vi "analyse.vi"(8 "error in (no error)":errorcluster, 11 "TrajectoryDL091126GenericVoxel in":refnum<class "TrajectoryDL091126GenericVoxel.lvclass">) -> (0 "error out":errorcluster, 3 "TrajectoryDL091126GenericVoxel out":refnum<class "TrajectoryDL091126GenericVoxel.lvclass">)   [LabVIEW 2010, in "TrajectoryDL091126GenericVoxel.lvclass"]
uses:
  TrajectoryDL091126GenericVoxel.lvclass
  common/classes/ImageCollection/ImageCollection/ImageCollection.lvclass
  common/enumerations/x_y_z_enumeration.ctl
  common/enumerations/functional_global_action_enum.ctl
  common/classes/ImageCollection/ImageCollection/add_mode_enum.ctl
  common/classes/Image/Image/Image.lvclass
  common/classes/ErrorController/ErrorController/class_data.vi
  <vilib>/vision/NI_Vision_Development_Module.lvlib
  common/classes/ErrorController/ErrorController/ErrorController.lvclass
panel:
  in  "loadZPositionDataButton":bool
  in  "loadYPositionDataButton":bool
  out "y signals 2":dbl[][](graph)
  in  "position scale z":dbl(slide) scale=0.0..20000.0
  in  "position scale y":dbl(slide) scale=0.0..20000.0
  out "y signals":dbl[][](graph)
  in  "position scale x":dbl(slide) scale=0.0..20000.0
  in  "defineTrajectoryButton":bool
  in  "line":i32(slide) scale=0.0..10.0
  out "x signals":dbl[][](graph)
  in  "doneButton":bool
  in  "loadXPositionDataButton":bool
  # "Analyse position feedback"
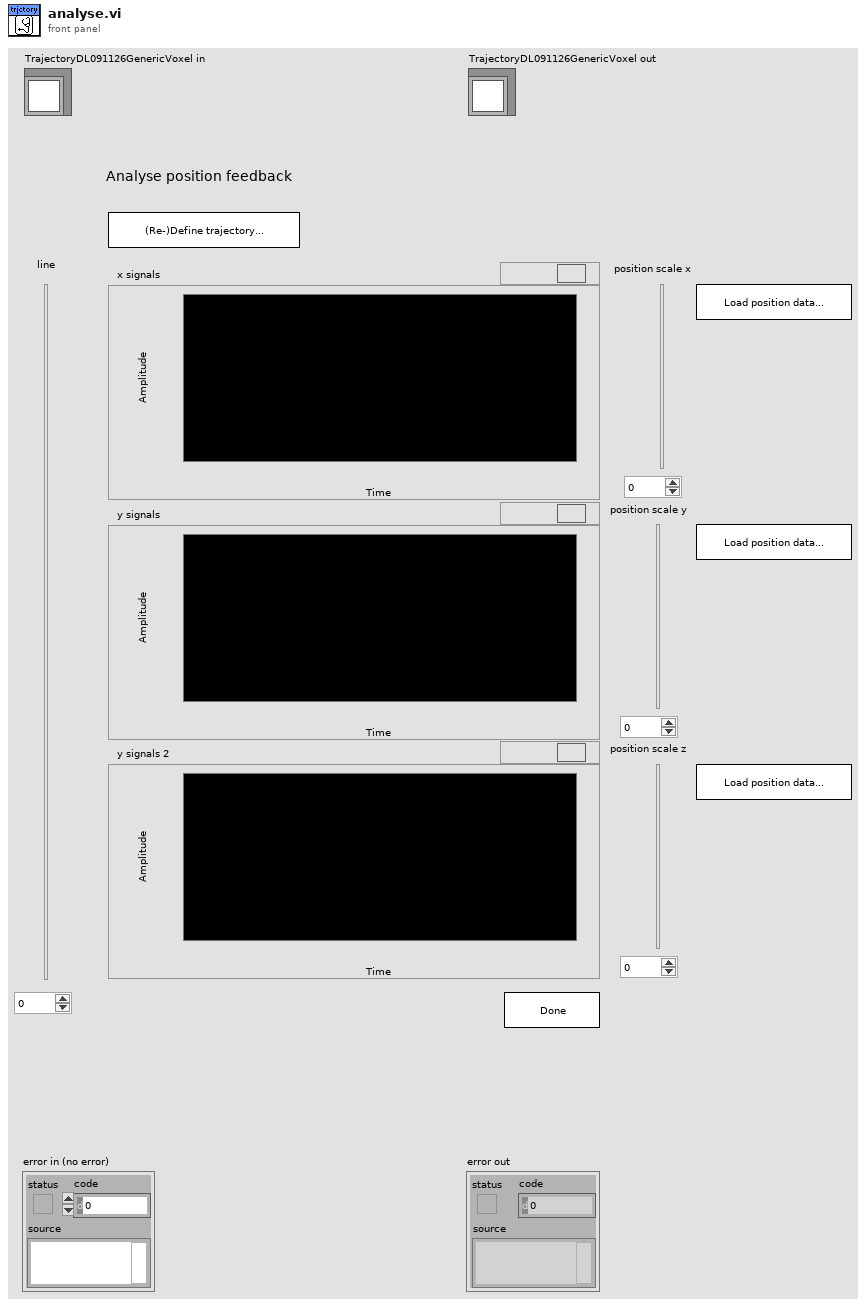
[diagram p1: front panel]
types:
  T1 = typedef "x_y_z_enumeration.ctl" = enum16{"x", "y", "z"}
  T2 = typedef "Image Type" = u32
  T3 = typedef "functional_global_action_enum.ctl" = enum16{"get", "set", "reset"}
  T4 = typedef "ImageCollection.lvclass/add_mode_enum.ctl" = enum16{"instance", "copy"}
  T5 = typedef "IMAQ Image.ctl" = refnum<image>
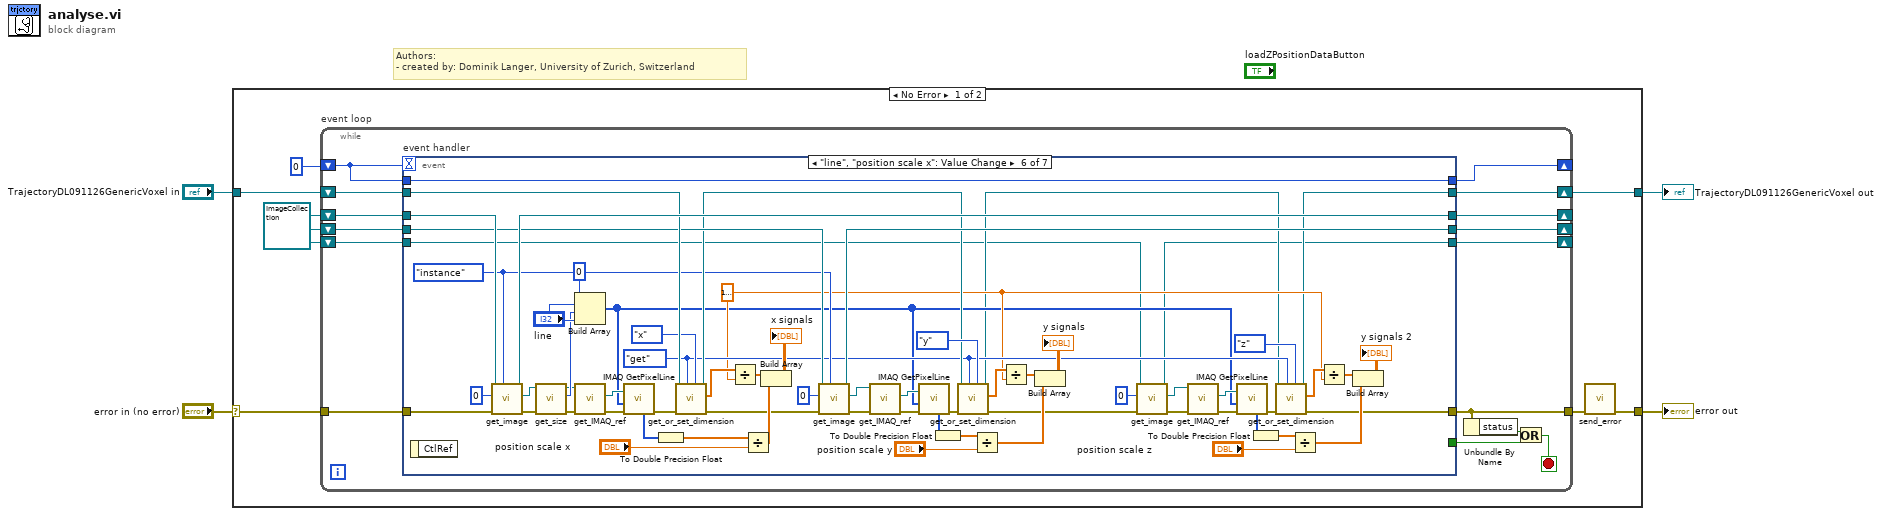
[diagram p0: block diagram]
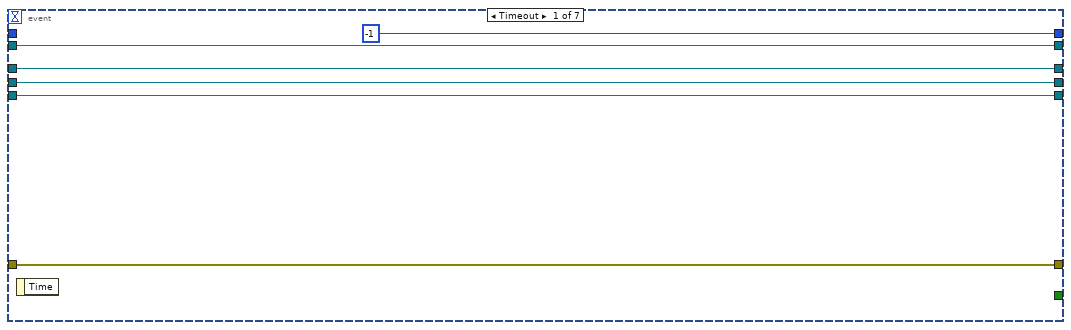
[diagram p2: hidden frame]
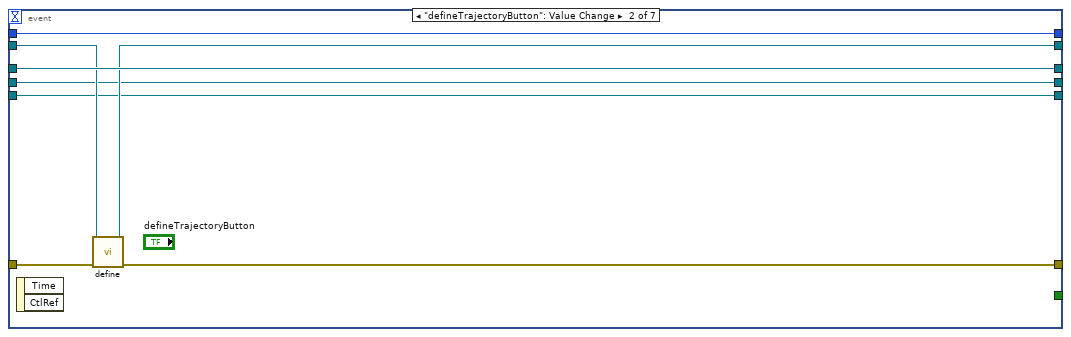
[diagram p3: hidden frame]
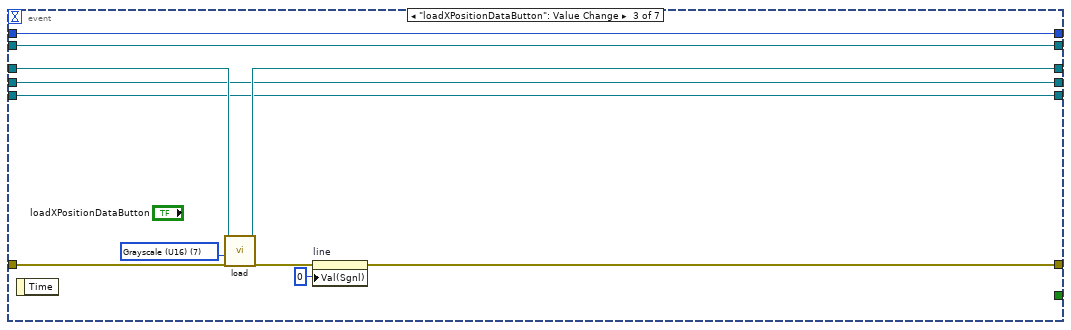
[diagram p4: hidden frame]
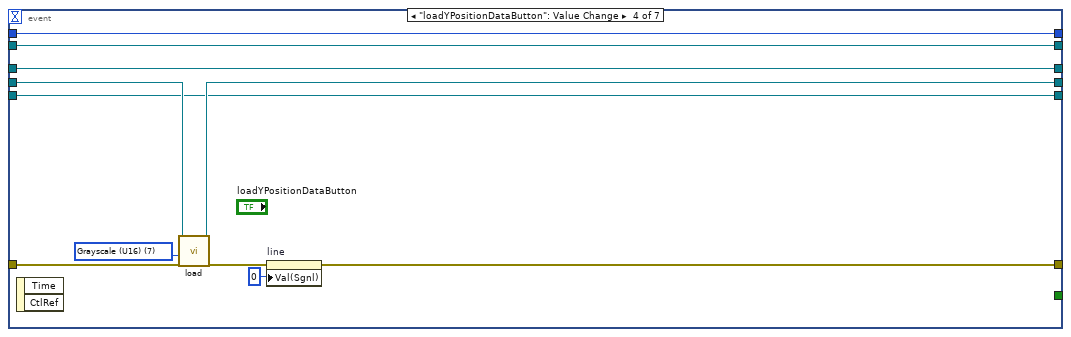
[diagram p5: hidden frame]
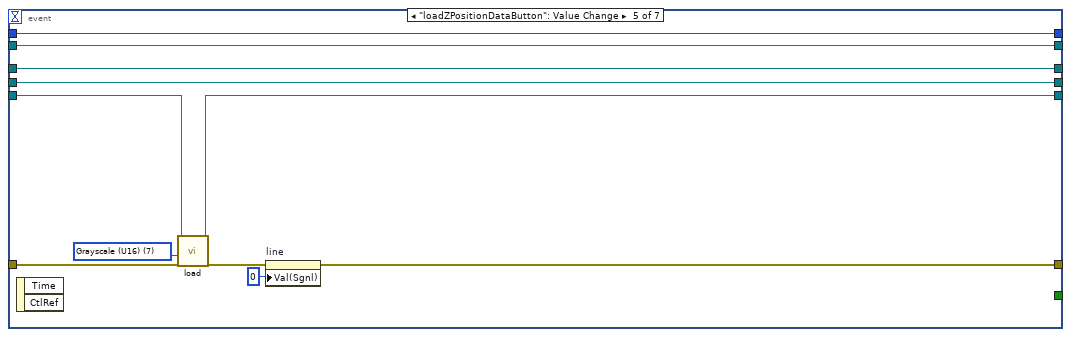
[diagram p6: hidden frame]
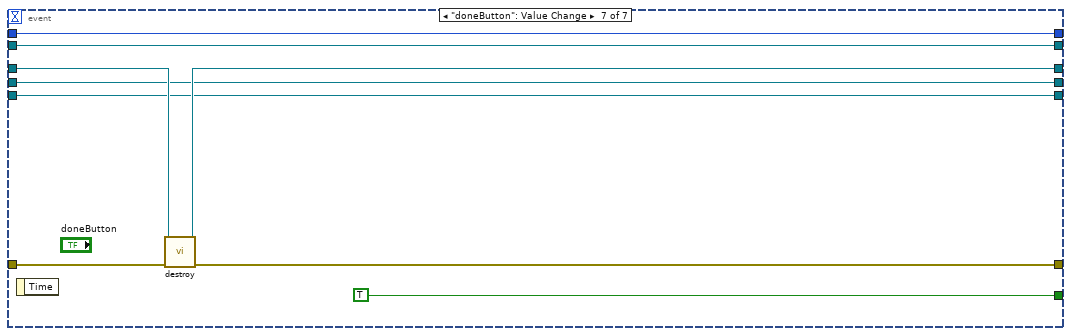
[diagram p7: hidden frame]
diagram:
  # "Authors: \n- created by: Dominik Langer, University of Zurich, Switzerland"
  n1 = case shown="No Error" "error in (no error)" {
    selector: "error in (no error)" -> [w11 w150]
    tunnel: [w5 w150] -> w3
    tunnel: [w9 w149] -> w1
    tunnel: "TrajectoryDL091126GenericVoxel in" -> [w10 w149]
    frame No Error {
      w7 = refnum<class "ImageCollection.lvclass"> refnum ("ImageCollection.lvclass")
      n2 = while "event loop" {
        shift-right: [w25] -> w9
        shift-left: w10 -> [w26]
        shift-right: [w18] -> _
        shift-left: w7 -> [w19]
        shift-right: [w16] -> _
        shift-left: 0 -> [w17]
        shift-right: [w13] -> _
        shift-left: w7 -> [w15]
        shift-right: [w12] -> _
        shift-left: w7 -> [w14]
        tunnel: w11 -> [w24]
        tunnel: [w23] -> w6
        stop <- w22 stop-if-true
        n3 = event "event handler" shown="[5] \"line\", \"position scale x \": Value Change" {
          selector: _ -> [_ _ _ _ _ _ _]
          dyn-events: _ -> [_ _ _ _ _ _ _]
          timeout: w17 -> [_ _ _ _ _ _ _]
          tunnel: w26 -> [w32 w36 w51 w62 w73 w124 w148]
          tunnel: [w32 w35 w51 w62 w73 w76 w148] -> w25
          tunnel: w24 -> [w29 w39 w50 w55 w64 w139 w144]
          tunnel: [w29 w38 w45 w54 w63 w82 w143] -> w23
          tunnel: [_ _ _ _ _ _ TRUE] -> w21
          tunnel: [w30 w37 w48 w61 w72 w136 w145] -> w18
          tunnel: w19 -> [w30 w37 w49 w61 w72 w137 w146]
          tunnel: [-1 w40 w43 w60 w71 w126 w142] -> w16
          tunnel: w17 -> [_ w40 w43 w60 w71 w126 w142]
          tunnel: w15 -> [w28 w34 w42 w56 w70 w108 w141]
          tunnel: w14 -> [w27 w33 w41 w52 w66 w75 w140]
          tunnel: [w28 w34 w42 w53 w70 w107 w141] -> w13
          tunnel: [w27 w33 w41 w52 w65 w74 w140] -> w12
          event Timeout {
            n4 = event-data() -> ()  [unwired: 1 in, 1 out]
          }
          event "defineTrajectoryButton": Value Change {
            n5 = event-data() -> ()  [unwired: 1 in, 2 out]
            n6 = call-dynamic "define.vi"("error in (no error)"=w39, "GenericTrajectory in"=w36) -> ("error out"=w38:errorcluster, "GenericTrajectory out"=w35:refnum<class "TrajectoryDL091126GenericVoxel.lvclass">)  [unwired: 8 in]
          }
          event "loadXPositionDataButton": Value Change {
            w47 = T2 7 items=["Grayscale (U8)", "Grayscale (I16)", "Grayscale (SGL)", "Complex (CSG)", "RGB (U32)", "HSL (U32)", "RGB (U64)", "Grayscale (U16)"] ("Image Type")
            n7 = event-data() -> ()  [unwired: 1 in, 1 out]
            n8 = call "load.vi"("error in (no error)"=w50, "Image Type"=w47, "ImageCollection in"=w49) -> ("error out"=w46:errorcluster, "ImageCollection out"=w48:refnum<class "ImageCollection.lvclass">)  [unwired: 4 in, 3 out]
            n9 = property on="line" class="Slide (strict)"(error in=w46, "Val(Sgnl)"=0 ("Value (Signaling)")) -> (error out=w45:errorcluster)  [unwired: 1 in, 1 out]
          }
          event "loadYPositionDataButton": Value Change {
            w59 = T2 7 items=["Grayscale (U8)", "Grayscale (I16)", "Grayscale (SGL)", "Complex (CSG)", "RGB (U32)", "HSL (U32)", "RGB (U64)", "Grayscale (U16)"] ("Image Type")
            n10 = event-data() -> ()  [unwired: 1 in, 2 out]
            n11 = call "load.vi"("error in (no error)"=w55, "Image Type"=w59, "ImageCollection in"=w56) -> ("error out"=w58:errorcluster, "ImageCollection out"=w53:refnum<class "ImageCollection.lvclass">)  [unwired: 4 in, 3 out]
            n12 = property on="line" class="Slide (strict)"(error in=w58, "Val(Sgnl)"=0 ("Value (Signaling)")) -> (error out=w54:errorcluster)  [unwired: 1 in, 1 out]
          }
          event "loadZPositionDataButton": Value Change {
            w67 = T2 7 items=["Grayscale (U8)", "Grayscale (I16)", "Grayscale (SGL)", "Complex (CSG)", "RGB (U32)", "HSL (U32)", "RGB (U64)", "Grayscale (U16)"] ("Image Type")
            n13 = event-data() -> ()  [unwired: 1 in, 2 out]
            n14 = call "load.vi"("error in (no error)"=w64, "Image Type"=w67, "ImageCollection in"=w66) -> ("error out"=w68:errorcluster, "ImageCollection out"=w65:refnum<class "ImageCollection.lvclass">)  [unwired: 4 in, 3 out]
            n15 = property on="line" class="Slide (strict)"(error in=w68, "Val(Sgnl)"=0 ("Value (Signaling)")) -> (error out=w63:errorcluster)  [unwired: 1 in, 1 out]
          }
          event "line", "position scale x": Value Change {
            w80 = dbl[unit] 1e-06 ("Numeric")
            w81 = functional_global_action_enum."get" ("action")
            w101 = add_mode_enum."instance" ("get image as...")
            n16 = event-data() -> ()  [unwired: 1 in, 1 out]
            n17 = call-dynamic "get_image.vi"("get image as..."=w101, "error in (no error)"=w139, "index"=0, "ImageCollection in"=w137) -> ("error out"=w131:errorcluster, "Image.lvclass"=w129:refnum<class "Image.lvclass">, "ImageCollection out"=w136:refnum<class "ImageCollection.lvclass">)  [unwired: 5 in]
            n18 = call-dynamic "get_size.vi"("error in (no error)"=w131, "Image in"=w129) -> ("error out"=w130:errorcluster, "x resolution"=w128:i32, "Image out"=w127:refnum<class "Image.lvclass">)  [unwired: 2 in, 5 out]
            n19 = Build Array(0, "line", w128, "line") -> (w79:i32[])
            n20 = call-dynamic "get_IMAQ_ref.vi"("error in (no error)"=w130, "Image.lvclass in"=w127) -> ("error out"=w135:errorcluster, "Image"=w134:T5)  [unwired: 5 in, 3 out]
            n21 = call "IMAQ GetPixelLine"("error in (no error)"=w135, "Line Coordinates"=w79, "Image"=w134) -> ("Pixels Line (U16)"=w122:u16[], "error out"=w125:errorcluster)  [unwired: 1 in, 3 out]
            n22 = To Double Precision Float(number=w122) -> (double precision float=w118:dbl[])
            n23 = call-dynamic "get_or_set_dimension.vi"("dimension"=x_y_z_enumeration."x", "action"=w81, "error in (no error)"=w125, "GenericTrajectory in"=w124) -> ("error out"=w109:errorcluster, "pixel values out (single dimension)"=w121:dbl[unit][], "GenericTrajectory out"=w106:refnum<class "TrajectoryDL091126GenericVoxel.lvclass">)  [unwired: 5 in]
            n24 = Divide(x=w121, y=w80) -> (x/y=w120:dbl[])
            n25 = Divide(x=w118, y="position scale x") -> (x/y=w117:dbl[])
            n26 = Build Array(w120, w117) -> (→"x signals":dbl[][])
            n27 = call-dynamic "get_image.vi"("get image as..."=w101, "error in (no error)"=w109, "index"=0, "ImageCollection in"=w108) -> ("error out"=w103:errorcluster, "Image.lvclass"=w102:refnum<class "Image.lvclass">, "ImageCollection out"=w107:refnum<class "ImageCollection.lvclass">)  [unwired: 5 in]
            n28 = call-dynamic "get_IMAQ_ref.vi"("error in (no error)"=w103, "Image.lvclass in"=w102) -> ("error out"=w111:errorcluster, "Image"=w113:T5)  [unwired: 5 in, 3 out]
            n29 = call "IMAQ GetPixelLine"("error in (no error)"=w111, "Line Coordinates"=w79, "Image"=w113) -> ("Pixels Line (U16)"=w100:u16[], "error out"=w110:errorcluster)  [unwired: 1 in, 3 out]
            n30 = To Double Precision Float(number=w100) -> (double precision float=w99:dbl[])
            n31 = call-dynamic "get_or_set_dimension.vi"("dimension"=x_y_z_enumeration."y", "action"=w81, "error in (no error)"=w110, "GenericTrajectory in"=w106) -> ("error out"=w83:errorcluster, "pixel values out (single dimension)"=w115:dbl[unit][], "GenericTrajectory out"=w77:refnum<class "TrajectoryDL091126GenericVoxel.lvclass">)  [unwired: 5 in]
            n32 = Divide(x=w99, y="position scale y") -> (x/y=w97:dbl[])
            n33 = Divide(x=w115, y=w80) -> (x/y=w105:dbl[])
            n34 = Build Array(w105, w97) -> (→"y signals":dbl[][])
            n35 = call-dynamic "get_image.vi"("error in (no error)"=w83, "index"=0, "ImageCollection in"=w75) -> ("error out"=w91:errorcluster, "Image.lvclass"=w92:refnum<class "Image.lvclass">, "ImageCollection out"=w74:refnum<class "ImageCollection.lvclass">)  [unwired: 6 in]
            n36 = call-dynamic "get_IMAQ_ref.vi"("error in (no error)"=w91, "Image.lvclass in"=w92) -> ("error out"=w87:errorcluster, "Image"=w85:T5)  [unwired: 5 in, 3 out]
            n37 = call "IMAQ GetPixelLine"("error in (no error)"=w87, "Line Coordinates"=w79, "Image"=w85) -> ("Pixels Line (U16)"=w93:u16[], "error out"=w88:errorcluster)  [unwired: 1 in, 3 out]
            n38 = To Double Precision Float(number=w93) -> (double precision float=w94:dbl[])
            n39 = call-dynamic "get_or_set_dimension.vi"("dimension"=x_y_z_enumeration."z", "action"=w81, "error in (no error)"=w88, "GenericTrajectory in"=w77) -> ("error out"=w82:errorcluster, "pixel values out (single dimension)"=w84:dbl[unit][], "GenericTrajectory out"=w76:refnum<class "TrajectoryDL091126GenericVoxel.lvclass">)  [unwired: 5 in]
            n40 = Divide(x=w94, y="position scale z") -> (x/y=w96:dbl[])
            n41 = Divide(x=w84, y=w80) -> (x/y=w89:dbl[])
            n42 = Build Array(w89, w96) -> (→"y signals 2":dbl[][])
          }
          event "doneButton": Value Change {
            n43 = event-data() -> ()  [unwired: 1 in, 1 out]
            n44 = call-dynamic "destroy.vi"("error in (no error)"=w144, "ImageCollection in"=w146) -> ("error out"=w143:errorcluster, "ImageCollection out"=w145:refnum<class "ImageCollection.lvclass">)  [unwired: 8 in]
          }
        }
        n45 = Unbundle By Name(w23) -> ("status"=w20:bool)
        n46 = Or(x=w20, y=w21) -> (x .or. y?=w22:bool)
      }
      n47 = call "send_error.vi"("error in (no error)"=w6) -> ("error out"=w5:errorcluster)  [unwired: 10 in]
    }
    frame Error {
    }
  }
  "error out" <- w3
  "TrajectoryDL091126GenericVoxel out" <- w1
